vi "unregisterEvent.vi"(8 "error in (no error)":errorcluster, 10 "Event Callback in":refnum<k27>, 11 "SM1000-control in":T1) -> (0 "error out":errorcluster, 3 "SM1000-control out":T1)   [LabVIEW 2013, in "MaterialCharacterization.lvlib" / "MC-SM1000.lvclass"]
doc: "Unregisters the application for 'OnConnect'-events."
uses:
  MC-SM1000.lvclass
  Object-reference.ctl
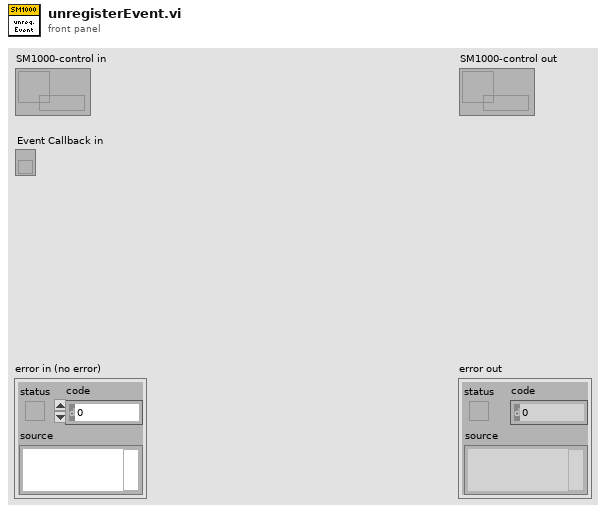
[diagram p1: front panel]
types:
  T1 = typedef "MaterialCharacterization.lvlib/MC-SM1000.lvclass/Object-reference.ctl" = refnum<data-value>
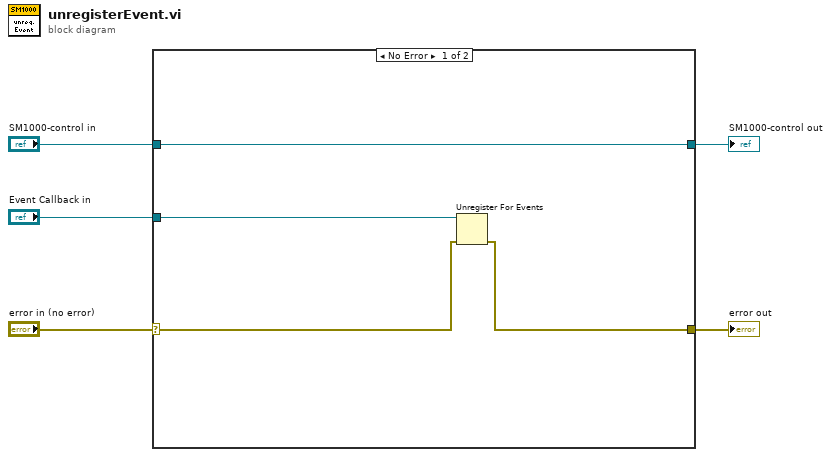
[diagram p0: block diagram]
diagram:
  n1 = case shown="No Error" "error in (no error)" {
    selector: "error in (no error)" -> [w7 w11]
    tunnel: [w6 w11] -> w4
    tunnel: [w9 w10] -> w2
    tunnel: "SM1000-control in" -> [w9 w10]
    tunnel: "Event Callback in" -> [w8 _]
    frame No Error {
      n2 = Unregister For Events(event registration refnum=w8, error in=w7) -> (error out=w6:errorcluster)
    }
    frame Error {
    }
  }
  "error out" <- w4
  "SM1000-control out" <- w2
